vi "Laser Test.vi"() -> ()   [LabVIEW 2022 SP3]
uses:
  <vilib>/MakerHub/LINX/Public/Utilities/Open Serial.vi
  <vilib>/MakerHub/LINX/LMH-LINX.lvlib
panel:
  out "Error Out":errorcluster
  out "Overheat":bool
  out "Energy":dbl(slide) scale=0.0..100.0
  in  "Trigger Pin":u8=3
  in  "Laser Pin":u8=6
  in  "Stop Button":bool
  in  "Serial Port":refnum<visa-resource-name>="N/A"
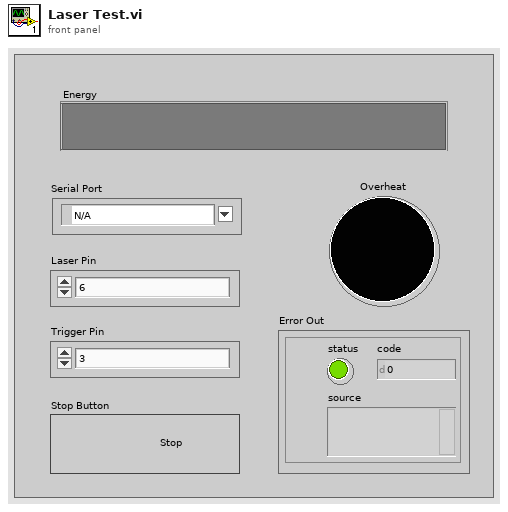
[diagram p1: front panel]
types:
  T1 = typedef "LMH-LINX.lvlib/LINX Ref.ctl" = cluster{"IO":T2, "Interface":T3, "LINX Device Config":T4}
  T2 = typedef "LMH-LINX.lvlib/Platform.ctl" = enum16{"Remote", "Local"}
  T3 = typedef "LMH-LINX.lvlib/Interface.ctl" = enum16{"Serial", "TCP"}
  T4 = typedef "LMH-LINX.lvlib/Device.lvlib/LINX Device Config.ctl" = cluster{"Interface":T3, "COM Port":refnum<visa-resource-name>, "TCP Configuration":T5, "Device Family":u8, "Device ID":u8, "Device Name":string, "TCP Ref":refnum<k5>, "Channels":T6}
  T5 = typedef "LMH-LINX.lvlib/Device.lvlib/TCP Config.ctl" = cluster{"IP Address":string, "Port":u16}
  T6 = typedef "LMH-LINX.lvlib/Channels.ctl" = cluster{"DI":u8[], "DO":u8[], "AI":u8[], "AO":u8[], "PWM":u8[], "QE":u8[], "UART":u8[], "I2C 2":u8[], "SPI":u8[], "CAN":u8[], "Servo":u8[], "AI Ref (V)":dbl, "AI Resolution (Bits)":u8, "AO Ref (V)":dbl, "AO Resolution (Bits)":u8}
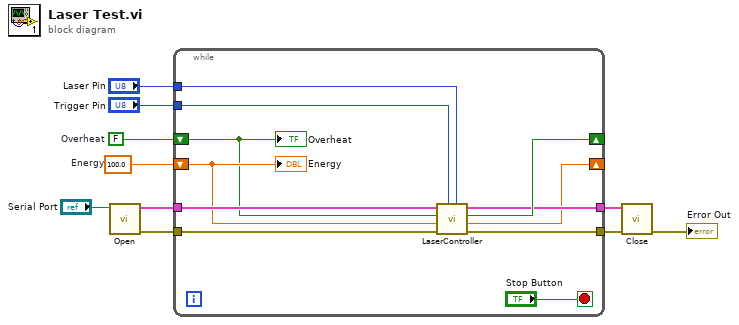
[diagram p0: block diagram]
diagram:
  w5 = FALSE  # Overheat
  w6 = 100.0  # Energy
  n1 = call-poly <vilib>:"Open.vi"("Serial Port"="Serial Port") -> ("Error Out"=w9:errorcluster, "LINX Resource"=w10:T1)  [unwired: 8 in, 1 out]
  n2 = while {
    tunnel: w10 -> [w17]
    tunnel: w9 -> [w20]
    tunnel: "Laser Pin" -> [w19]
    tunnel: "Trigger Pin" -> [w18]
    shift-right: [w11] -> _
    shift-left: w6 -> [w14]
    shift-right: [w16] -> _
    shift-left: w5 -> [w13]
    tunnel: [w15] -> w2
    tunnel: [w12] -> w1
    stop <- "Stop Button" stop-if-true
    n3 = call "LaserController.vi"("Laser Pin"=w19, "Trigger Pin"=w18, "Error In"=w20, "Energy In"=w14, "Overheat In"=w13, "LINX Resource In"=w17) -> ("Error Out"=w15:errorcluster, "Energy Out"=w11:dbl, "Overheat Out"=w16:bool, "LINX Resource Out"=w12:T1)  [unwired: 2 in]
    "Energy" <- w14
    "Overheat" <- w13
  }
  n4 = call <vilib>:"Close.vi"("Error In"=w2, "LINX Resource"=w1) -> ("Error Out"=→"Error Out":errorcluster)  [unwired: 9 in]
